vi "Scan_BU2.vi"(0 "DMM ref":refnum<visa-resource-name>, 1 "channel_count":i32=11, 2 "P_current_count":i32, 3 "N_current_count":i32, 5 "DMM error":errorcluster, 9 "ESP32 ref":refnum<visa-resource-name>, 11 "ESP32 error":errorcluster, 12 "current_mode":u8[](array[numeric])=[0, 0, 0, 0, 0, 0, 0, 0, 0, 0, 0]) -> (4 "DMM ref":refnum<visa-resource-name>, 6 "DMM error":errorcluster, 8 "Measurements":dbl[](array[numeric]), 10 "ESP32 ref":refnum<visa-resource-name>, 13 "Timout?":bool, 14 "Time out count":i32, 15 "ESP32 error":errorcluster)   [LabVIEW 2023]
uses:
  <instrlib>/Agilent 3446X Series/Agilent 3446X Series.lvlib
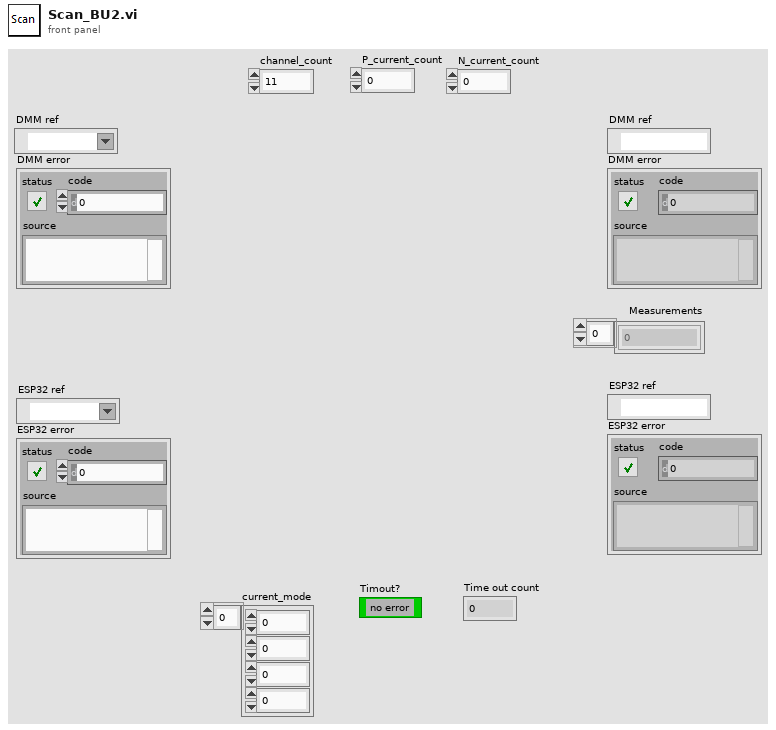
[diagram p1: front panel]
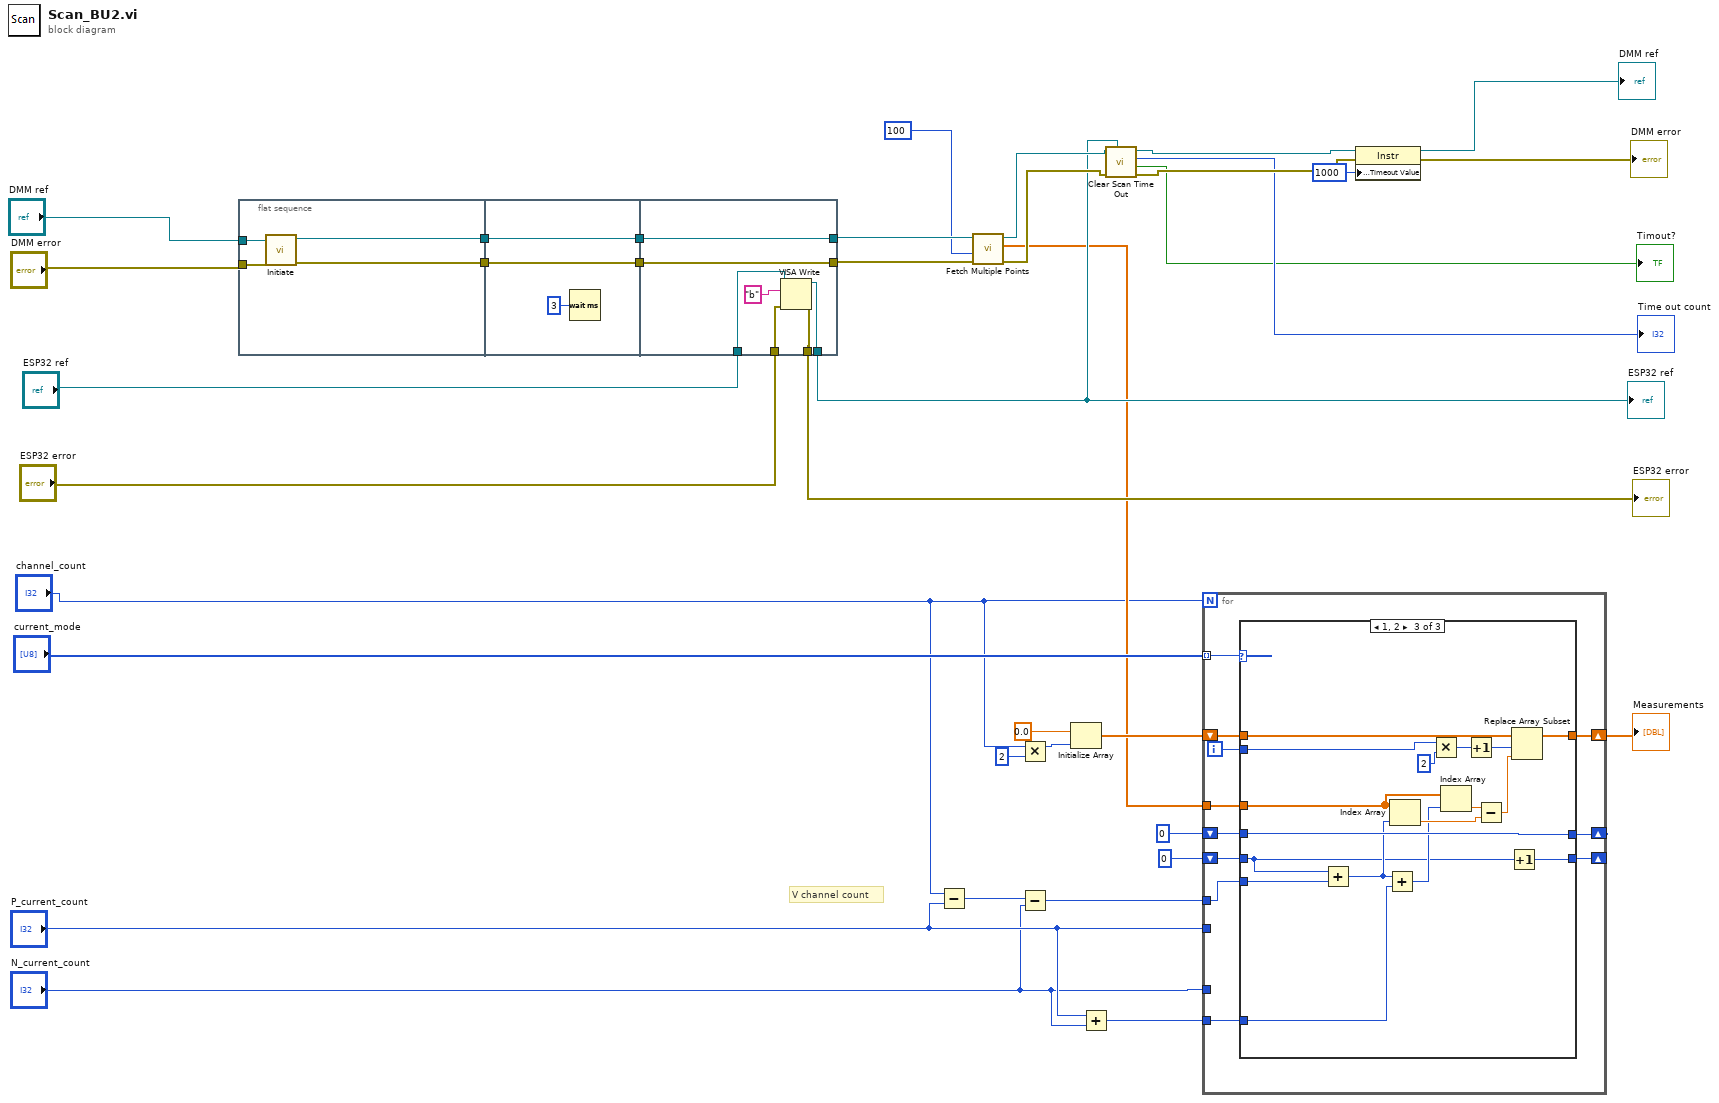
[diagram p0: block diagram]
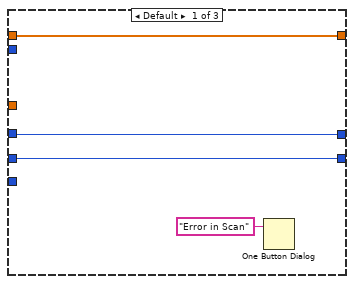
[diagram p2: hidden frame]
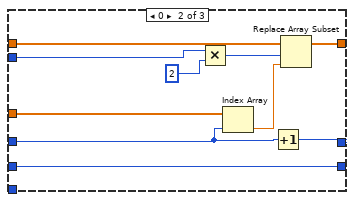
[diagram p3: hidden frame]
diagram:
  # "V channel count"
  n1 = flat-sequence {
    tunnel: [w41] -> w37
    tunnel: [w40] -> w36
    tunnel: "DMM ref" -> [w39]
    tunnel: "DMM error" -> [w38]
    tunnel: w37 -> [w44]
    tunnel: [w44] -> w35
    tunnel: w36 -> [w43]
    tunnel: [w43] -> w34
    tunnel: w35 -> [w51]
    tunnel: w34 -> [w50]
    tunnel: "ESP32 ref" -> [w49]
    tunnel: "ESP32 error" -> [w48]
    tunnel: [w47] -> w18
    tunnel: [w46] -> w19
    tunnel: [w51] -> w33
    tunnel: [w50] -> w32
    frame #0 {
      n2 = call <instrlib>:"Initiate.vi"("error in (no error)"=w38, "VISA resource name"=w39) -> ("error out"=w41:errorcluster, "VISA resource name out"=w40:refnum<visa-resource-name>)  [unwired: 8 in]
    }
    frame #1 {
      n3 = Wait (ms)(milliseconds to wait=u32 3) -> ()  [unwired: 1 out]
    }
    frame #2 {
      n4 = VISA Write(VISA resource name=w49, write buffer="b" ("data in"), error in (no error)=w48) -> (VISA resource name out=w47:refnum<visa-resource-name>, error out=w46:errorcluster)  [unwired: 1 out]
    }
  }
  n5 = Subtract(x="channel_count", y="P_current_count") -> (x-y=w8:i32)
  n6 = call <instrlib>:"Fetch Multiple Points.vi"("error in (no error)"=w33, "Timeout (10000 ms)"=100, "VISA resource name"=w32) -> ("error out"=w28:errorcluster, "Measurements"=w10:dbl[], "VISA resource name out"=w29:refnum<visa-resource-name>)  [unwired: 1 in, 5 out]
  n7 = Multiply(x="channel_count", y=2) -> (x*y=w14:i32)
  n8 = Subtract(x=w8, y="N_current_count") -> (x-y=w7:i32)
  n9 = Initialize Array(0.0 ("Measurement"), w14) -> (w12:dbl[])
  n10 = Add(x="P_current_count", y="N_current_count") -> (x+y=w2:i32)
  n11 = call "Clear Scan Time Out.vi"("ESP32 ref"=w18, "error in (no error)"=w28, "VISA Refnum in"=w29) -> ("error out"=w26:errorcluster, "error?"=→"Timout?":bool, "Time out count"=→"Time out count":i32, "VISA Refnum out"=w27:refnum<visa-resource-name>)  [unwired: 5 in]
  n12 = for {
    N: "channel_count" -> [_]
    shift-right: [w56] -> w1
    shift-left: w12 -> [w57]
    tunnel: "current_mode" -> [w62] mode=indexing
    tunnel: w10 -> [w61]
    tunnel: "P_current_count" -> [_]
    tunnel: "N_current_count" -> [_]
    tunnel: w7 -> [w53]
    shift-right: [w59] -> _
    shift-left: 0 ("index") -> [w60]
    shift-right: [w54] -> _
    shift-left: 0 ("index") -> [w55]
    tunnel: w2 -> [w52]
    i -> [w58]
    n13 = case shown="1, 2" w62 {
      tunnel: w61 -> [_ w76 w86]
      tunnel: w60 -> [w66 w74 w87]
      tunnel: [w66 w73 w87] -> w59
      tunnel: w58 -> [_ w71 w92]
      tunnel: w57 -> [w65 w72 w93]
      tunnel: [w65 w69 w89] -> w56
      tunnel: w55 -> [w64 w68 w78]
      tunnel: [w64 w68 w77] -> w54
      tunnel: w53 -> [_ _ w82]
      tunnel: w52 -> [_ _ w81]
      frame Default {
        n14 = One Button Dialog(message="Error in Scan") -> ()  [unwired: 1 in, 1 out]
      }
      frame 0 {
        n15 = Multiply(x=w71, y=2 ("x")) -> (x*y=w67:i32)
        n16 = Index Array(array=w76, index=w74) -> (element=w75:dbl)
        n17 = Increment(x=w74) -> (x+1=w73:i32)
        n18 = Replace Array Subset(array=w72, new element=w75, index=w67) -> (w69:dbl[])
      }
      frame 1, 2 {
        n19 = Add(x=w78, y=w82) -> (x+y=w80:i32)
        n20 = Add(x=w80, y=w81) -> (x+y=w79:i32)
        n21 = Index Array(array=w86, index=w80) -> (element=w84:dbl)
        n22 = Multiply(x=w92, y=2 ("x")) -> (x*y=w90:i32)
        n23 = Index Array(array=w86, index=w79) -> (element=w85:dbl)
        n24 = Increment(x=w90) -> (x+1=w88:i32)
        n25 = Subtract(x=w85, y=w84) -> (x-y=w83:dbl)
        n26 = Increment(x=w78) -> (x+1=w77:i32)
        n27 = Replace Array Subset(array=w93, new element=w83, index=w88) -> (w89:dbl[])
      }
    }
  }
  "Measurements" <- w1
  n28 = property class="Instr"(reference=w27, error in=w26, "General Settings:Timeout Value"=u32 1000) -> (reference out=→"DMM ref":refnum<visa-resource-name>, error out=→"DMM error":errorcluster)
  "ESP32 ref" <- w18
  "ESP32 error" <- w19
